vi "CompareTrackerBias.vi"() -> ()   [LabVIEW 2011]
uses:
  qtrk/QTrkLVBinding/XYZf.ctl
  qtrk/lv/CPUTrkAPI.llb/TrackerDLL.vi
panel:
  out "Radial profile":dbl[](graph)
  out "LV XCor":dbl[](graph)
  out "Image":sgl[][](graph)
  out "Array":dbl[](array[numeric])
  out "LV QI":dbl[](graph)
  out "QTrk QI":dbl[](graph)
  out "iteration":i32
  in  "X Range":dbl=4.0
  out "Intensity Graph":dbl[][](graph)
  in  "tracker DLL path":path=path "D:/jcnossen1/cudaqi-tracker/qtrk/lv/qtrk-labview.dll"
  in  "# images":i32=1000
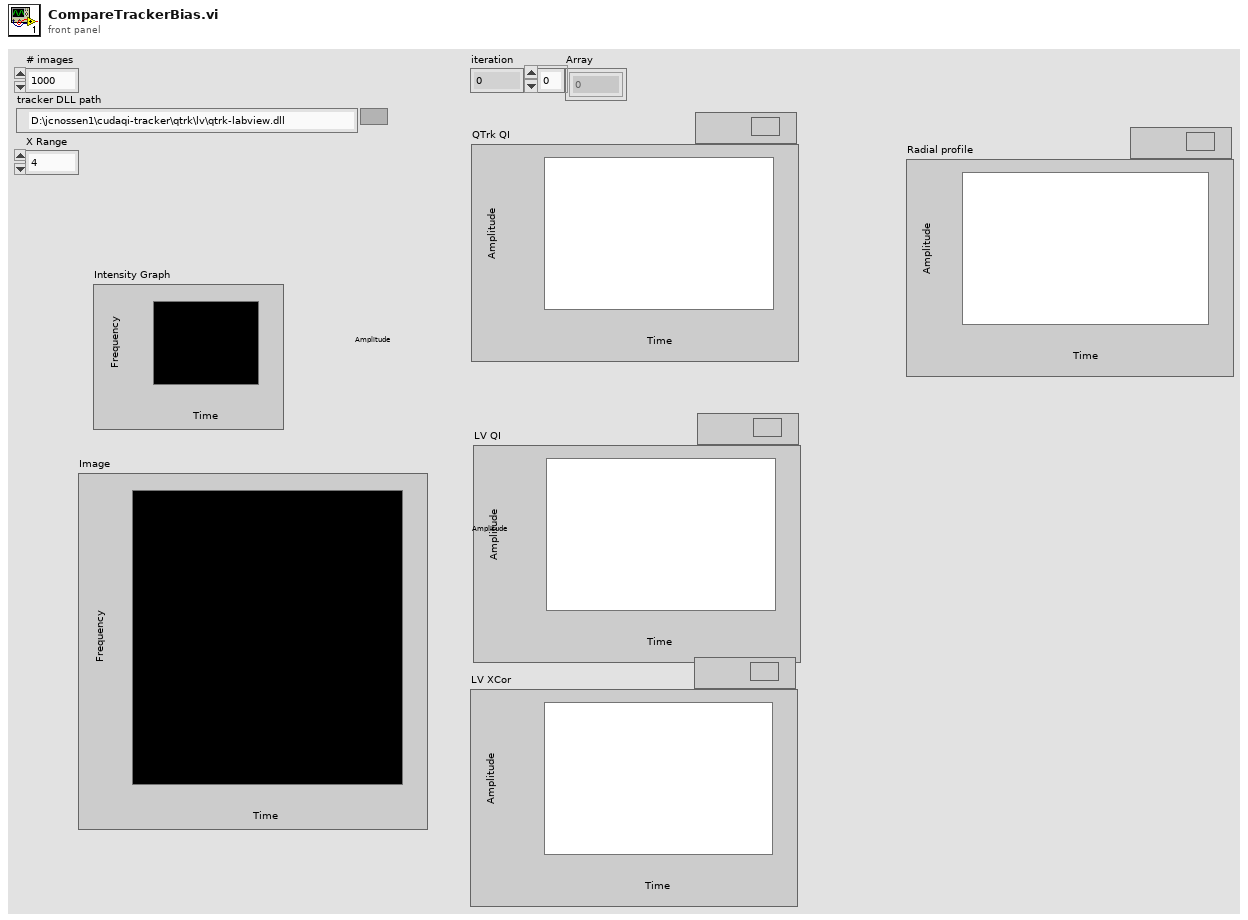
[diagram p1: front panel]
types:
  T1 = typedef "TrackerInstance.ctl" = cluster{"Tracker Pointer":u64, "Image size":cluster{"width":u32, "height":u32}}
  T2 = cluster{"Rmax (pix)":i32, "RminZ (pix)":i32, "angular pixel\n coverage factor":dbl, "radial pixel\n coverage factor":dbl}
  T3 = typedef "XYZf.ctl" = cluster{"X":sgl, "Y":sgl, "Z":sgl}
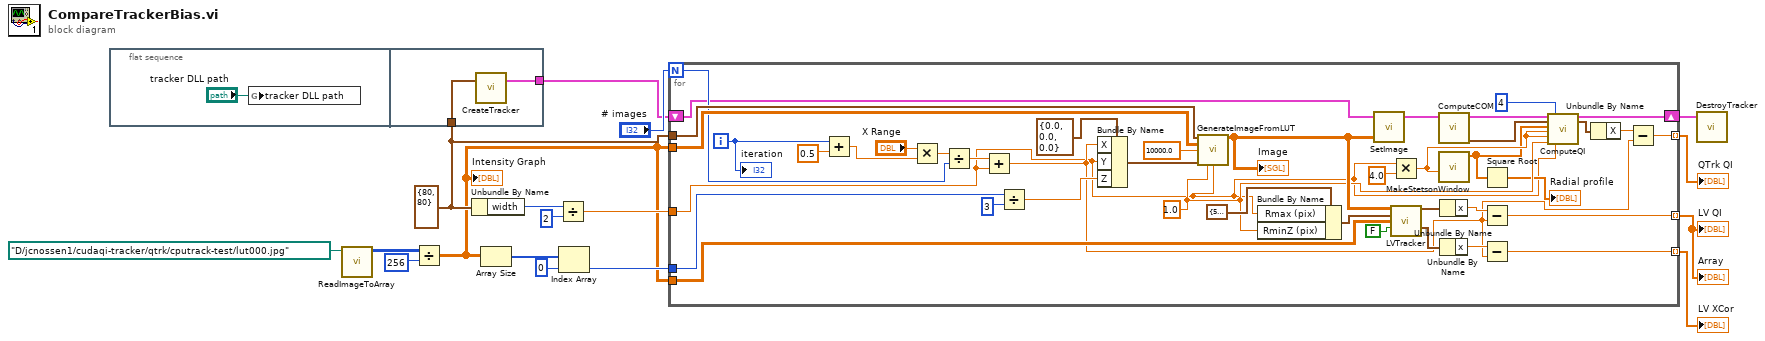
[diagram p0: block diagram]
diagram:
  w12 = cluster{"width":u32, "height":u32} {"width"=80, "height"=80} ("Image size")
  n1 = flat-sequence {
    tunnel: [w20] -> w16
    tunnel: w12 -> [w19]
    frame #0 {
      n2 = global write "TrackerDLL.vi" "tracker DLL path"("tracker DLL path") -> ()
    }
    frame #1 {
      n3 = call "CreateTracker.vi"("Image size"=w19) -> ("tracker"=w20:T1)  [unwired: 2 in]
    }
  }
  n4 = call "ReadImageToArray.vi"("File Path"=path "D:/jcnossen1/cudaqi-tracker/qtrk/cputrack-test/lut000.jpg") -> ("Image Pixels (U8)"=w14:u8[][])  [unwired: 7 in, 3 out]
  n5 = Divide(x=w14, y=256 ("# images")) -> (x/y=w4:dbl[][])
  "Intensity Graph" <- w4
  n6 = Unbundle By Name(w12) -> ("width"=w11:u32)
  n7 = Array Size(array=w4) -> (size(s)=w8:i32[])
  n8 = Divide(x=w11, y=u32 2) -> (x/y=w9:dbl)
  n9 = Index Array(array=w8, index=0) -> (element=w6:i32)
  n10 = for {
    N: "# images" -> [w57]
    tunnel: w12 -> [w62]
    tunnel: w4 -> [w61]
    tunnel: w9 -> [w22]
    tunnel: w6 -> [w50]
    shift-right: [w42] -> w2
    shift-left: w16 -> [w51]
    tunnel: [w30] -> w5 mode=indexing
    tunnel: w4 -> [w40]
    tunnel: [w32] -> w3 mode=indexing
    tunnel: [w26] -> w1 mode=indexing
    i -> [w56]
    w34 = sgl 1.0 ("minRadius")
    n11 = Add(x=w56, y=0.5 ("X Range")) -> (x+y=w54:dbl)
    n12 = Multiply(x="X Range", y=w54) -> (x*y=w58:dbl)
    n13 = Divide(x=w58, y=w57) -> (x/y=w52:dbl)
    n14 = Add(x=w52, y=w22) -> (x+y=w27:dbl)
    n15 = Divide(x=w50, y=3) -> (x/y=w48:dbl)
    n16 = Bundle By Name(cluster=T3 {"X"=0.0, "Y"=0.0, "Z"=0.0} ("XYZ"), "X"=w27, "Y"=w22, "Z"=w48) -> (w47:T3)
    n17 = call "GenerateImageFromLUT.vi"("Image Size"=w62, "ZLUT"=w61, "Pixel max value"=sgl 10000.0, "XYZ"=w47, "ZLUT MinRadius"=w34, "ZLUT MaxRadius"=w22) -> ("Result image"=w35:sgl[][])  [unwired: 9 in]
    "Image" <- w35
    n18 = Bundle By Name(cluster=T2 {"Rmax (pix)"=50, "RminZ (pix)"=5, "angular pixel\n coverage factor"=0.7, "radial pixel\n coverage factor"=3.0} ("settings"), "Rmax (pix)"=w22, "RminZ (pix)"=w34) -> (w37:T2)
    n19 = call "SetImage.vi"("tracker"=w51, "Image (float)"=w35) -> ("tracker"=w46:T1)  [unwired: 6 in, 1 out]
    n20 = Multiply(x=w22, y=4.0) -> (x*y=w24:dbl)
    n21 = call "LVTracker.vi"("image in"=w35, "settings"=w37, "Z LUT"=w40, "Compute Z"=FALSE) -> ("qi position"=w36:cluster{"x":dbl, "y":dbl}, "xcor position"=w29:cluster{"x":dbl, "y":dbl})  [unwired: 6 in, 4 out]
    n22 = call "ComputeCOM.vi"("tracker"=w46) -> ("position"=w44:cluster{"X":sgl, "Y":sgl}, "tracker"=w45:T1)  [unwired: 5 in]
    n23 = call "MakeStetsonWindow.vi"("radialsteps"=w24) -> ("Window"=w21:dbl[])  [unwired: 10 in]
    n24 = Unbundle By Name(w36) -> ("x"=w33:dbl)
    n25 = Unbundle By Name(w29) -> ("x"=w28:dbl)
    n26 = Square Root(x=w21) -> (sqrt(x)=→"Radial profile":dbl[])
    n27 = Subtract(x=w33, y=w27) -> (x-y=w32:dbl)
    n28 = Subtract(x=w28, y=w27) -> (x-y=w26:dbl)
    n29 = call "ComputeQI.vi"("tracker"=w45, "initial position"=w44, "radial weights (such as stetson window)"=w21, "radialSteps"=w24, "angularStepsPerQuadrant"=w24, "minRadius"=w34, "iterations"=4, "maxRadius"=w22) -> ("tracker"=w42:T1, "position"=w41:cluster{"X":sgl, "Y":sgl})  [unwired: 9 in, 1 out]
    n30 = Unbundle By Name(w41) -> ("X"=w31:sgl)
    n31 = Subtract(x=w31, y=w27) -> (x-y=w30:dbl)
    "iteration" <- w56
  }
  "QTrk QI" <- w5
  "LV QI" <- w3
  "Array" <- w3
  "LV XCor" <- w1
  n32 = call "DestroyTracker.vi"("tracker instance"=w2) -> ()  [unwired: 5 in]
